vi "class_data.vi"() -> ()   [LabVIEW 2010, in "GenericImageAssembler.lvclass"]
uses:
  GenericImageAssembler.lvclass
panel:
  in  "latest instance":refnum<class "GenericImageAssembler.lvclass">
  in  "locked by":string
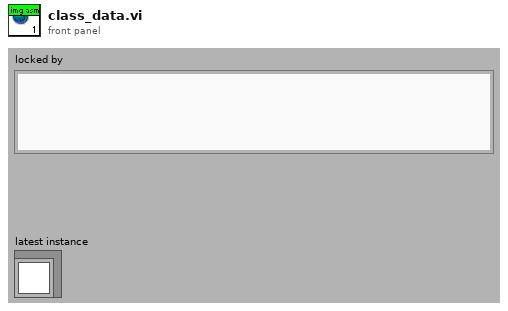
[diagram p1: front panel]
diagram:
